vi "PlantModel.vi"() -> ()   [LabVIEW 2015]
uses:
  <vilib>/Utility/miscctls.llb/LV3DPointTypeDef.ctl
  <vilib>/Simulation/Scripting/Companion Diagram/SimConfigNode/SimParams.ctl
  <vilib>/Simulation/Scripting/Companion Diagram/SimConfigNode/_simSolvers.ctl
  <vilib>/Simulation/Implementation/Shared/SIMSCR Execution Mode.ctl
  <vilib>/Simulation/Param Hierarchy/Typedefs/SIMPH Param Control Actions.ctl
  <vilib>/Simulation/Implementation/Shared/SIM limit type.ctl
  <vilib>/Simulation/Scripting/Editor Utilities/SIM subVI tag data.ctl
  <vilib>/Simulation/Scripting/Editor Utilities/SIM subVI execution type.ctl
  <vilib>/Simulation/Implementation/Shared/NILVSim_ParamChanged.vi
  <vilib>/Simulation/Implementation/Shared/NILVSIM_BeginStep.vi
  <vilib>/Simulation/Nonlinear/Implementation/NILVSim Quantizer.llb/SIM Quantizer (scalar).vi
  <vilib>/Simulation/Utility/Implementation/SIM Halt.vi
  <vilib>/Simulation/SignalArithmetic/Implementation/NILVSim Gain.llb/SIM Gain (vector).vi
  <vilib>/Simulation/SignalArithmetic/Implementation/NILVSim Gain.llb/SIM Gain (vector,MatrixGain).vi
  <vilib>/Simulation/ContinuousLinear/Implementation/NILVSim Integrator new.llb/SIM Integrator distributor (scalar).vi
  <vilib>/Simulation/SignalDisplay/Implementation/NILVSim Time Waveform.llb/SIM Time Waveform (scalar).vi
  <vilib>/Simulation/ContinuousLinear/Implementation/NILVSim Integrator new.llb/SIM Integrator collector (scalar).vi
  <vilib>/Simulation/Implementation/Shared/SIM Fire Discrete SubVI.vi
  <vilib>/Simulation/Implementation/Shared/NILVSim_Manager.vi
  <vilib>/Utility/error.llb/Clear Errors.vi
  <vilib>/Simulation/Implementation/Shared/NILVSim_FinalizeModel.vi
  <vilib>/Simulation/Implementation/Shared/SIM Fire Discrete SubVI (Core).vi
  <vilib>/Simulation/Implementation/Shared/SIM Unbundle Sim Info.vi
  <vilib>/Simulation/Implementation/Shared/NILVSim_Initialize.vi
  <vilib>/ptbypt/Signal Generation.llb/Gaussian White Noise PtByPt.vi
  Model 1 LQR Modified V1/subVIs/inpparam.vi
  Model 1 LQR Modified V1/subVIs/matgen.vi
  Model 1 LQR Modified V1/subVIs/sysparam.vi
  <vilib>/Simulation/Utility/Implementation/NILVSim Get Time and IsAcceptedStep.vi
  Model 1 LQR Modified V1/subVIs/angset.vi
  Model 1 LQR Modified V1/subVIs/cdex - update quadcopter 3D model.vi
  Model 1 LQR Modified V1/subVIs/input.vi
  Model 1 LQR Modified V1/subVIs/ssa.vi
  Model 1 LQR Modified V1/subVIs/battery.vi
  <vilib>/Simulation/Implementation/Shared/SIMSH Read Queue.vi
  <vilib>/Simulation/Implementation/Shared/NILVSim_GetModelError.vi
  <vilib>/Simulation/Implementation/Shared/SIM Bundle Sim Info.vi
  <vilib>/Simulation/Scripting/Companion Diagram/SimConfigNode/SimDog.xnode
  <vilib>/Simulation/Implementation/XNodeFramework/SimXNode/SimX.xnode
  <resource>/objmgr/ni.dex.rc
  <vilib>/Simulation/ContinuousLinear/Implementation/NILVSim Integrator new.llb/SIM Integrator (scalar).vi
  <vilib>/ptbypt/NI_PtbyPt.lvlib
  <vilib>/Simulation/Implementation/Shared/NI_SIM_Implementation.lvlib
panel:
  out "Expected":dbl[](array[numeric])
  out "data out":dbl[](array[numeric])
  out "Is Connected":bool
  out "RT reader URL 2":string
  out "3D Picture Control 3":refnum<vi>(3d-picture)
  in  "Longitude (Y)":dbl(slide) scale=0.0..10.0
  in  "Latitude (X)":dbl(slide)
  in  "Altitude (Z)":dbl(slide)=2.0 scale=0.0..10.0
  out "X":waveform(dbl)(graph)
  out "Y":waveform(dbl)(graph)
  out "Z":waveform(dbl)(graph)
  out "Phi":waveform(dbl)(graph)
  out "Theta":waveform(dbl)(graph)
  out "Psi":waveform(dbl)(graph)
  out "Yo":dbl[](array[numeric])
  out "A":dbl[][](array[numeric])
  out "B":dbl[][](array[numeric])
  in  "Environmental effects":dbl(slide) scale=0.0..100.0
  in  "Stop Button":bool
  out "Motors Speed":dbl[](array[slide]) scale=0.0..6000.0
  out "Present Current":dbl
  out "Present Voltage":dbl
  out "Current Usage":dbl
  out "Battery Percentage":dbl(slide) scale=0.0..100.0
  out "StateOut":dbl[](array[numeric])
  in  "myRIO IP address":string="172.22.11.2"
  out "RT reader URL":string
  out "RT connected?":bool
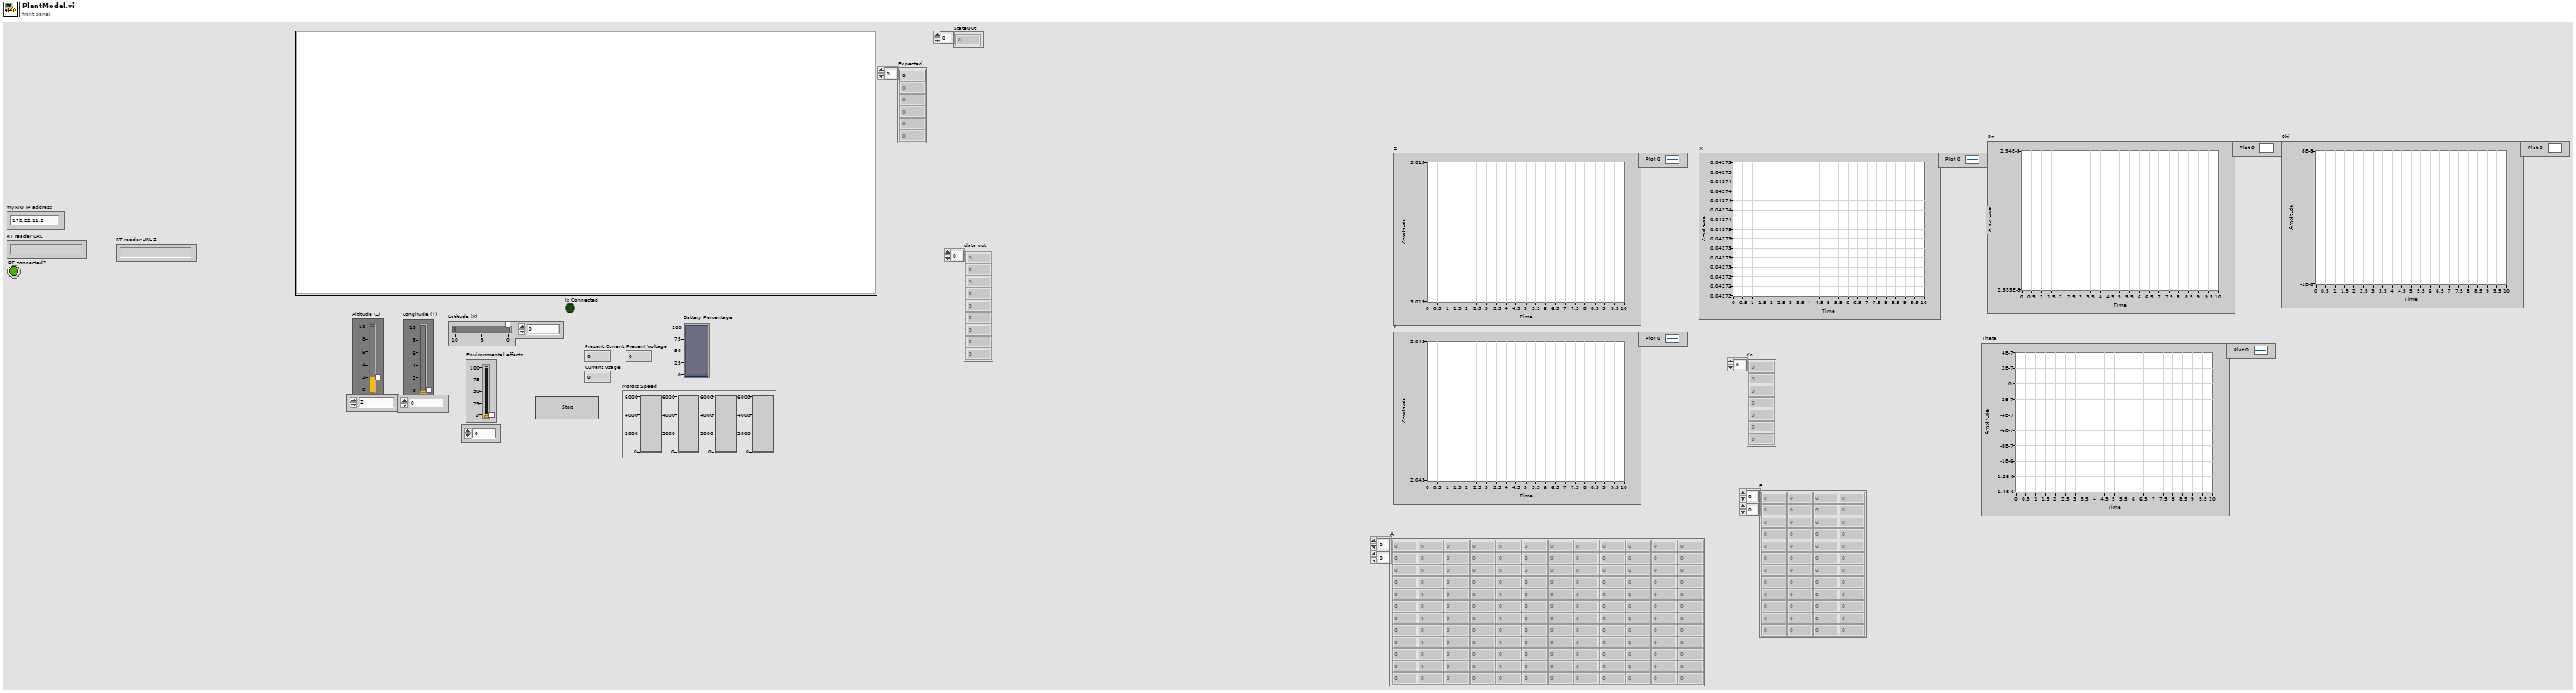
[diagram p1: front panel]
types:
  T1 = typedef "LV3DPointTypeDef.ctl" = cluster{"X":sgl, "Y":sgl, "Z":sgl}
  T2 = typedef "SIMSCR Execution Mode.ctl" = enum16{"Simulate to Completion", "Single Time-Step Simulation (Fixed Step Only)"}
  T3 = typedef "SIMPH Param Control Actions.ctl" = enum16{"get params", "set params"}
  T4 = typedef "SIM subVI tag data.ctl" = cluster{"period":dbl, "skew":dbl, "Simulation execution type":T5}
  T5 = typedef "SIM subVI execution type.ctl" = enum16{"Function call", "Discrete", "Continuous", "Initialization only", "Final step only"}
  T6 = typedef "SIM limit type.ctl" = enum16{"upper", "lower", "both", "none"}
  T7 = typedef "SimParams.ctl" = cluster{"Initial Time (s)":dbl, "Final Time (s)":dbl, "Step Size (s)":dbl, "ODE Solver":T8, "Minimum Step Size (s)":dbl, "Maximum Step Size (s)":dbl, "Relative Tolerance":dbl, "Absolute Tolerance":dbl, "Software Timing":bool, "Initial Step Size (s)":dbl, "Automatic Fixed Step Size?":bool, "Automatic Discrete Step Size?":bool, "Discrete Step Size (s)":dbl, "Calculate using Time Step":bool, "Solver Wired?":bool, "Prev.Frm.Expected End":u64, "Prev.Frm.Actual End":u64, "Prev.Frm.Finished Late?":bool, "Prev.Iter.Expected End":u64, "Prev.Iter.Actual End":u64, "Prev.Iter.Finished Late?":bool, "Expected Iteration Start":u64, "Actual Iteration Start":u64, "Expected Frame Start":u64, "Actual Frame Start":u64, "Source Name":string, "Name":string, "Period":i64, "Deadline":i64, "Offset":i64, "Start":i64, "Priority":i32, "Timeout":i32, "Processor":i32, "Mode":enum32{"No Change", "Process missed periods, maintain original phase", "Discard missed periods, maintain original phase", "Process missed periods, ignore original phase", "Discard missed periods, ignore original phase"}, "Wakeup reason":enum32{"Normal", "Aborted", "Asynchronous wakeup", "Timing source error", "Timed loop error", "Timeout"}, "Error":errorcluster, "Source Type":string, "Secondary Source Type":string, "Global End Time":u64, "Global Start Time":u64, "Full Solver Reset":bool, "Execution Mode":T2, "Nan/Inf Check":bool, "Custom Solver Library":string, "Solver Is Variable":bool, "custom solver name":string, "Signal Collection Decimation":u32}
  T8 = typedef "_simSolvers.ctl" = enum16{"Runge-Kutta 1 (Euler)", "Runge-Kutta 2", "Runge-Kutta 3", "Runge-Kutta 4", "Runge-Kutta 23 (variable)", "Runge-Kutta 45 (variable)", "BDF (variable)", "Adams-Moulton (variable)", "Rosenbrock (variable)", "Discrete States Only", "SDIRK 4 (variable)", "Radau 5 (variable)", "Radau 9 (variable)", "Radau 13 (variable)", "Radau [Variable Order] (variable)", "Gear's Method (variable)", "Linearizer", "State Query", "Trim Eval", "Custom Solver"}
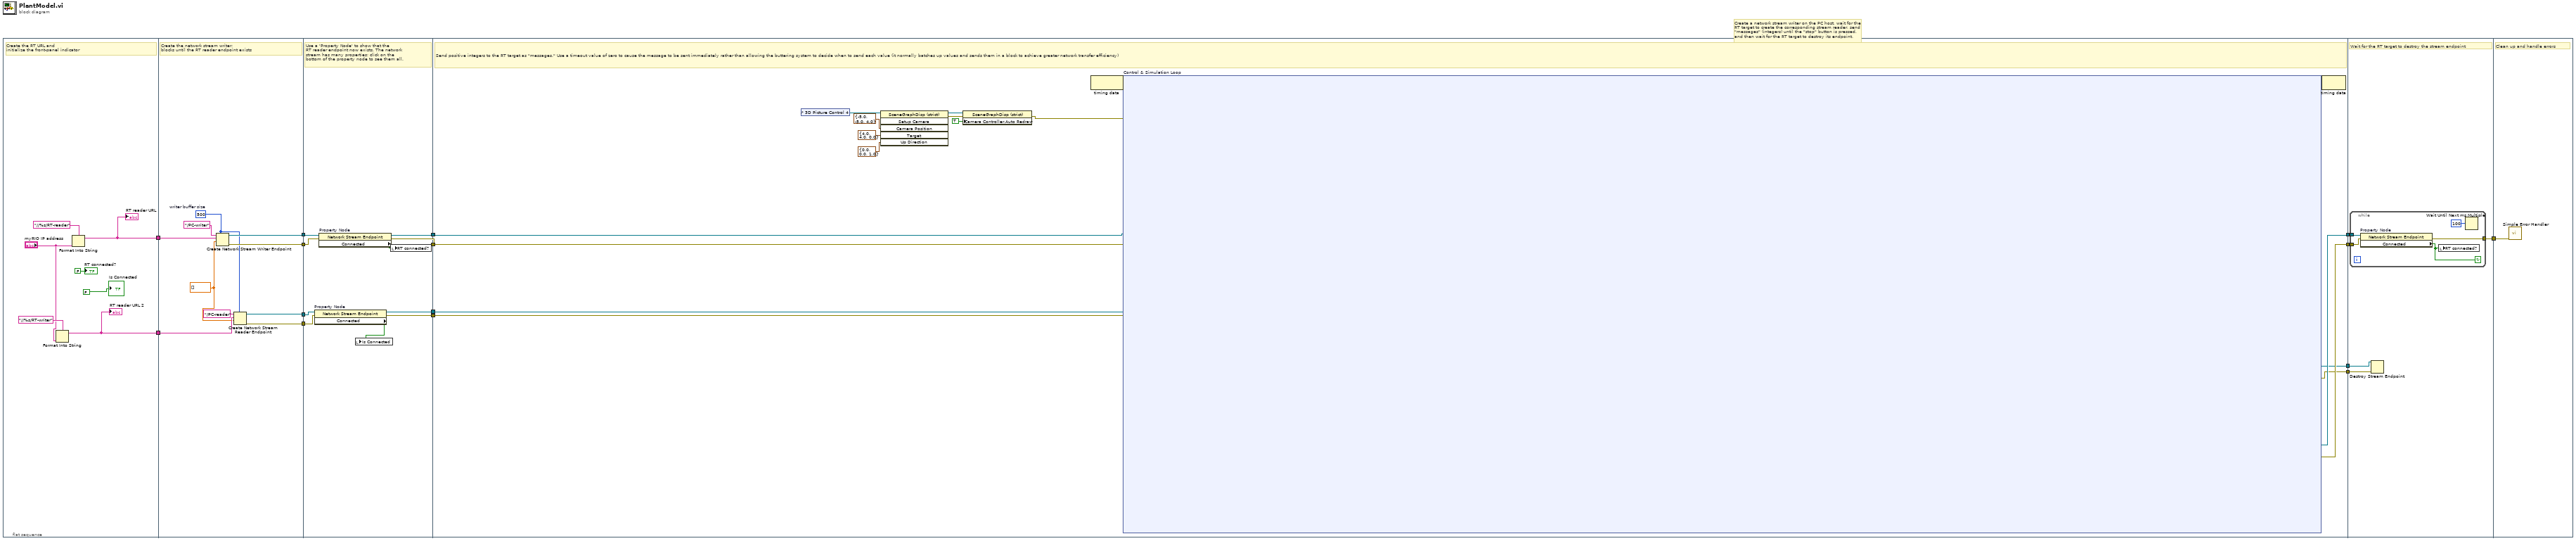
[diagram p0: block diagram]
diagram:
  # "Create a network stream writer on the PC host, wait for the\nRT target to create the corresponding stream reader, send\n\"messages\" (integers) until the \"stop\" button is pressed,\nand then wait for the RT target to destroy its endpoint."
  n1 = flat-sequence {
    tunnel: [w21] -> w15
    tunnel: [w17] -> w7
    tunnel: w15 -> [w31]
    tunnel: [w30] -> w14
    tunnel: [w29] -> w13
    tunnel: w7 -> [w28]
    tunnel: [w25] -> w6
    tunnel: [w24] -> w5
    tunnel: w14 -> [w42]
    tunnel: w13 -> [w41]
    tunnel: [w40] -> w12
    tunnel: [w39] -> w11
    tunnel: w6 -> [w37]
    tunnel: w5 -> [w36]
    tunnel: [w34] -> w4
    tunnel: [w33] -> w3
    tunnel: w12 -> [w56]
    tunnel: w11 -> [w55]
    tunnel: [w58] -> w9
    tunnel: [w57] -> w8
    tunnel: w4 -> [w46]
    tunnel: w3 -> [w45]
    tunnel: [w44] -> w2
    tunnel: [w43] -> w1
    tunnel: [w1221] -> w10
    tunnel: w9 -> [w1223]
    tunnel: w8 -> [w1222]
    tunnel: w2 -> [w1220]
    tunnel: w1 -> [w1219]
    tunnel: w10 -> [w1229]
    frame #0 {
      # "Create the RT URL and\ninitialize the front-panel indicator"
      n2 = Format Into String "Format Into String"(format string="//%s/RT-writer", "myRIO IP address") -> (resulting string=w17:string)  [unwired: 2 in, 1 out]
      "RT reader URL 2" <- w17
      n3 = Format Into String "Format Into String"(format string="//%s/RT-reader", "myRIO IP address") -> (resulting string=w21:string)  [unwired: 2 in, 1 out]
      "RT reader URL" <- w21
      "RT connected?" <- FALSE ("RT connected?")
      "Is Connected" <- FALSE ("RT connected?")
    }
    frame #1 {
      w26 = dbl[] [] ("Result")
      w23 = 500  # writer buffer size
      # "Create the network stream writer;\nblocks until the RT reader endpoint exists"
      n4 = Create Network Stream Writer Endpoint(7:w23, 9:w26, 10:w31, 11:"/PC-writer" ("writer name")) -> (0:w29:errorcluster, 3:w30:refnum<k21>)  [unwired: 3 in]
      n5 = Create Network Stream Reader Endpoint(7:w23, 9:w26, 10:w28, 11:"/PC-reader" ("reader name")) -> (0:w24:errorcluster, 3:w25:refnum<k21>)  [unwired: 3 in]
    }
    frame #2 {
      # "Use a 'Property Node' to show that the\nRT reader endpoint now exists. The network\nstream has many properties; click on the\nbottom of the property node to see them all."
      n6 = property on="Property Node" class="Network Stream Endpoint"(reference=w37, error in=w36) -> (reference out=w34:refnum<k21>, error out=w33:errorcluster, "Connected"=w35:bool)
      n7 = property on="Property Node" class="Network Stream Endpoint"(reference=w42, error in=w41) -> (reference out=w40:refnum<k21>, error out=w39:errorcluster, "Connected"=w38:bool)
      n8 = local write "Is Connected"(w35) -> ()
      n9 = local write "RT connected?"(w38) -> ()
    }
    frame #3 {
      # "Send positive integers to the RT target as \"messages.\" Use a timeout value of zero to cause the message to be sent immediately rather than allowing the buttering system to decide when to send each value (it normally batches up values and sends them in a block to achieve greater network transfer efficiency)"
      n10 = control-ref of="3D Picture Control 4"() -> (w54:refnum<vi>)
      n11 = invoke on="Invoke Node" class="SceneGraphDisp (strict)" method="Setup Camera"(reference=w54, "Camera Position"=T1 {"X"=-5.0, "Y"=-5.0, "Z"=4.0}, "Target"=T1 {"X"=4.0, "Y"=4.0, "Z"=0.0}, "Up Direction"=T1 {"X"=0.0, "Y"=0.0, "Z"=1.0}) -> (reference out=w52:refnum<vi>, error out=w53:errorcluster)  [unwired: 2 in, 4 out]
      n12 = property on="Property Node" class="SceneGraphDisp (strict)"(reference=w52, error in=w53, "Camera Controller.Auto Redraw"=TRUE ("Camera Controller:Auto Redraw")) -> (error out=w47:errorcluster)  [unwired: 1 out]
      n13 = node-c288() -> (w60:variant)  [unwired: 1 in]
      n14 = node-c254 "Control & Simulation Loop"(w60, w56, w55, w47, w46, w45) -> (w59:variant, w57:errorcluster, w58:refnum<k21>, w44:refnum<k21>, w43:errorcluster)
      n15 = node-c288(w59) -> ()  [unwired: 1 out]
    }
    frame #4 {
      # "Wait for the RT target to destroy the stream endpoint"
      n16 = while {
        tunnel: w1223 -> [w1228]
        tunnel: w1222 -> [w1227]
        tunnel: [w1226] -> w1221
        stop <- w1224 continue-if-true
        # "wait for RT to destroy the endpoint"
        n17 = property on="Property Node" class="Network Stream Endpoint"(reference=w1228, error in=w1227) -> (error out=w1226:errorcluster, "Connected"=w1224:bool)  [unwired: 1 out]
        n18 = local write "RT connected?"(w1224) -> ()
        n19 = Wait Until Next ms Multiple(millisecond multiple=u32 100) -> ()  [unwired: 1 out]
      }
      n20 = Destroy Stream Endpoint(8:w1219, 11:w1220) -> ()  [unwired: 1 out]
    }
    frame #5 {
      # "Clean up and handle errors"
      n21 = call <vilib>:"Simple Error Handler.vi"("error in (no error)"=w1229) -> ()  [unwired: 4 in, 5 out]
    }
  }
